vi "Read Attributes.vi"(11 "Check-Out Msg":refnum<class "Check-Out Msg.lvclass">) -> (2 "Payload":cluster{"Room No":string})   [LabVIEW 2023, in "Guest Manager UI.lvlib" / "Check-Out Msg.lvclass"]
uses:
  Check-Out Msg.lvclass
  Check-Out Msg.lvclass/Check-Out Msg.ctl
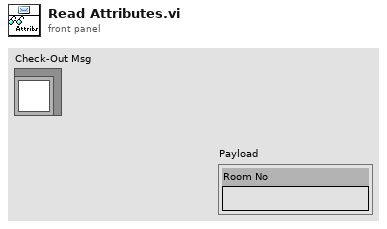
[diagram p1: front panel]
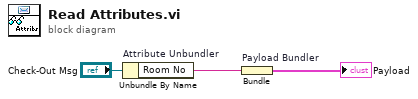
[diagram p0: block diagram]
diagram:
  n1 = Unbundle By Name "Attribute Unbundler"("Check-Out Msg") -> ("Room No"=w1:string)
  n2 = Bundle "Payload Bundler"("Room No"=w1) -> (→"Payload":cluster{"Room No":string})  [unwired: 1 in]
